vi "start.vi"(8 "error in (no error)":errorcluster, 9 "Parameters":T1, 10 "Model in":refnum<class "Model.lvclass">, 11 "StandbyState in":refnum<class "StandbyState.lvclass">) -> (0 "error out":errorcluster, 2 "Model out":refnum<class "Model.lvclass">, 3 "StandbyState out":refnum<class "StandbyState.lvclass">)   [LabVIEW 2016, in "StandbyState.lvclass"]
uses:
  StandbyState.lvclass
  Model/Model.lvclass
  DataTypes/Topics/CommandStart.ctl
  DataTypes/Topics/Parts/CommandId.ctl
  DataTypes/Topics/Parts/DetailedStates.ctl
  DataTypes/General/ILCModes.ctl
  DataTypes/Topics/M1M3SupportTopics.lvlib
  DataTypes/General/M1M3SupportGeneral.lvlib
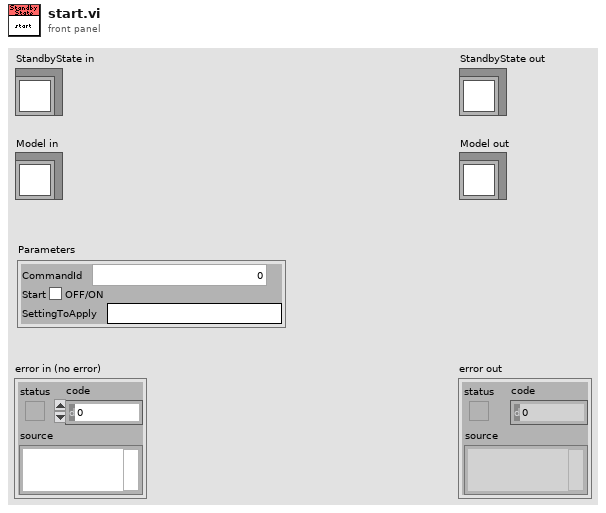
[diagram p1: front panel]
types:
  T1 = typedef "M1M3SupportTopics.lvlib/CommandStart.ctl" = cluster{"CommandId":T2, "Start":bool, "SettingToApply":string}
  T2 = typedef "M1M3SupportTopics.lvlib/CommandId.ctl" = i32
  T3 = typedef "M1M3SupportTopics.lvlib/DetailedStates.ctl" = enum16{"OfflineState", "InitialState", "StandbyState", "DisabledState", "ParkedState", "FaultState", "ParkedMaintenanceState", "ActiveMaintenanceState"}
  T4 = typedef "M1M3SupportGeneral.lvlib/ILCModes.ctl" = u16
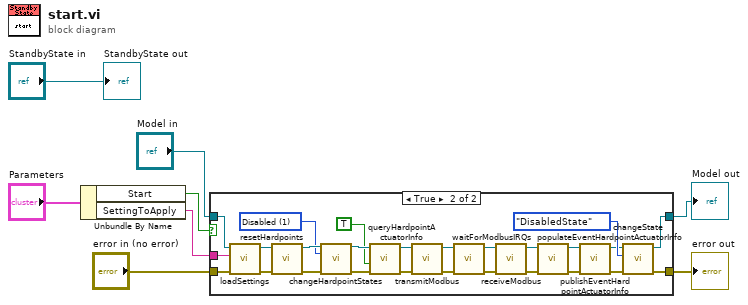
[diagram p0: block diagram]
diagram:
  n1 = Unbundle By Name("Parameters") -> ("Start"=w2:bool, "SettingToApply"=w1:string)
  n2 = case shown="True" w2 {
    tunnel: [w10 w36] -> w8
    tunnel: [w9 w35] -> w7
    tunnel: "Model in" -> [w10 w33]
    tunnel: "error in (no error)" -> [w9 w32]
    tunnel: w1 -> [_ w11]
    frame False {
    }
    frame True {
      w12 = T4 1 items=["Standby"=0, "Disabled"=1, "Enabled"=2, "FirmwareUpdate"=3, "Fault"=4, "Status"=65535] ("ILCModes")
      n3 = call "loadSettings.vi"("error in (no error)"=w32, "SettingToApply"=w11, "Model in"=w33) -> ("error out"=w22:errorcluster, "Model out"=w29:refnum<class "Model.lvclass">)  [unwired: 7 in]
      n4 = call "resetHardpoints.vi"("error in (no error)"=w22, "Model in"=w29) -> ("error out"=w21:errorcluster, "Model out"=w28:refnum<class "Model.lvclass">)  [unwired: 8 in]
      n5 = call "changeHardpointStates.vi"("Model in"=w28, "Mode"=w12, "error in (no error)"=w21) -> ("Model out"=w27:refnum<class "Model.lvclass">, "error out"=w20:errorcluster)  [unwired: 11 in]
      n6 = call "queryHardpointActuatorInfo.vi"("error in (no error)"=w20, "TriggerIRQ"=TRUE, "Model in"=w27) -> ("error out"=w19:errorcluster, "Model out"=w26:refnum<class "Model.lvclass">)  [unwired: 7 in]
      n7 = call "transmitModbus.vi"("error in (no error)"=w19, "Model in"=w26) -> ("error out"=w18:errorcluster, "Model out"=w25:refnum<class "Model.lvclass">)  [unwired: 8 in]
      n8 = call "waitForModbusIRQs.vi"("error in (no error)"=w18, "Model in"=w25) -> ("error out"=w17:errorcluster, "Model out"=w24:refnum<class "Model.lvclass">)  [unwired: 8 in]
      n9 = call "receiveModbus.vi"("error in (no error)"=w17, "Model in"=w24) -> ("error out"=w16:errorcluster, "Model out"=w23:refnum<class "Model.lvclass">)  [unwired: 8 in]
      n10 = call "populateEventHardpointActuatorInfo.vi"("error in (no error)"=w16, "Model in"=w23) -> ("error out"=w15:errorcluster, "Model out"=w31:refnum<class "Model.lvclass">)  [unwired: 8 in]
      n11 = call "publishEventHardpointActuatorInfo.vi"("error in (no error)"=w15, "Model in"=w31) -> ("error out"=w14:errorcluster, "Model out"=w30:refnum<class "Model.lvclass">)  [unwired: 8 in]
      n12 = call "changeState.vi"("error in (no error)"=w14, "DetailedStates"=DetailedStates."DisabledState", "Model in"=w30) -> ("error out"=w35:errorcluster, "Model out"=w36:refnum<class "Model.lvclass">)  [unwired: 7 in]
    }
  }
  "error out" <- w7
  "Model out" <- w8
  "StandbyState out" <- "StandbyState in"
